vi "MAP.vi"() -> ()   [LabVIEW 2014]
panel:
  in  "File Path":path
  out "Image":T1(plugin-control)
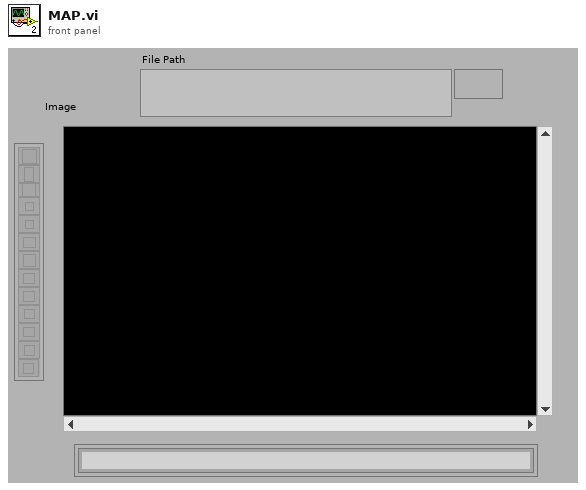
[diagram p1: front panel]
types:
  T1 = typedef "IMAQ Image.ctl" = refnum<image>
  T2 = typedef "Image Type" = u32
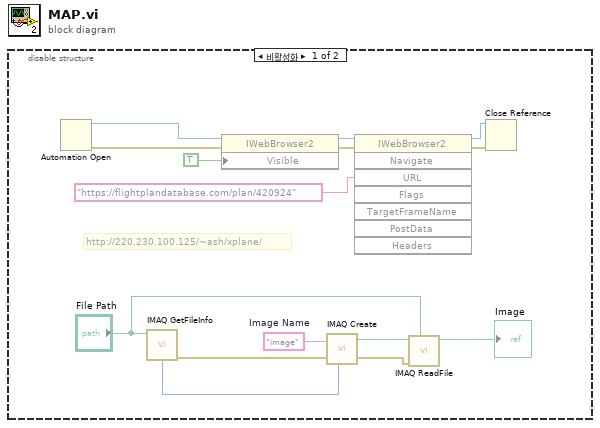
[diagram p0: block diagram]
diagram:
  n1 = disable-structure shown="비활성화" {
    frame Disabled {
      w1 = "image"  # Image Name
      # "http://220.230.100.125/~ash/xplane/"
      n2 = Automation Open() -> (Automation Refnum=w12:refnum<k7>, error out=w11:errorcluster)  [unwired: 2 in, 2 out]
      n3 = call "IMAQ GetFileInfo"("File Path"="File Path") -> ("error out"=w3:errorcluster, "Image Type"=w2:T2)  [unwired: 4 in, 5 out]
      n4 = property class="IWebBrowser2"(reference=w12, error in=w11, "Visible"=TRUE) -> (reference out=w13:refnum<k7>, error out=w14:errorcluster)
      n5 = call "IMAQ Create"("Image Name"=w1, "Image Type"=w2, "error in (no error)"=w3) -> ("New Image"=w4:T1, "error out"=w5:errorcluster)  [unwired: 2 in]
      n6 = invoke class="IWebBrowser2" method="Navigate"(reference=w13, error in=w14, "URL"="https://flightplandatabase.com/plan/420924") -> (reference out=w9:refnum<k7>, error out=w10:errorcluster)  [unwired: 5 in, 6 out]
      n7 = call "IMAQ ReadFile"("File Path"="File Path", "error in (no error)"=w5, "Image"=w4) -> ("Image Out"=→"Image":T1)  [unwired: 4 in, 4 out]
      n8 = Close Reference(reference=w9, error in (no error)=w10) -> ()  [unwired: 1 out]
    }
    frame Enabled {
    }
  }
